vi "swerve math.vi"() -> ()   [LabVIEW 2020]
panel:
  out "Back Right":cluster{"X":dbl, "Y":dbl}[](graph)
  out "Back Left":cluster{"X":dbl, "Y":dbl}[](graph)
  out "Front Right":cluster{"X":dbl, "Y":dbl}[](graph)
  in  "RCW":dbl(slide) scale=-1.0..1.0
  in  "STR":dbl(slide) scale=-1.0..1.0
  in  "FWD":dbl(slide) scale=-1.0..1.0
  out "Front Left":cluster{"X":dbl, "Y":dbl}[](graph)
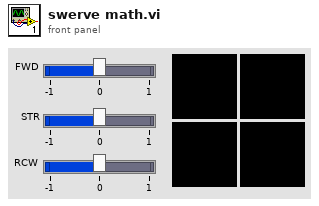
[diagram p1: front panel]
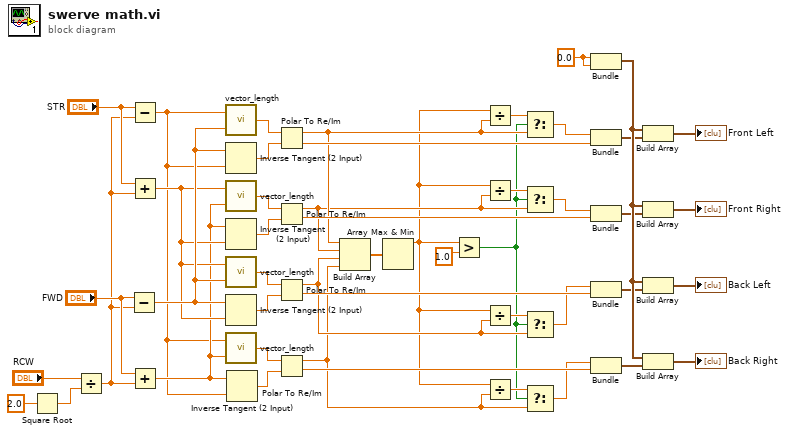
[diagram p0: block diagram]
diagram:
  w26 = 0.0 ("x")
  n1 = Square Root(x=2.0) -> (sqrt(x)=w48:dbl)
  n2 = Divide(x="RCW", y=w48) -> (x/y=w43:dbl)
  n3 = Subtract(x="FWD", y=w43) -> (x-y=w42:dbl)
  n4 = Subtract(x="STR", y=w43) -> (x-y=w39:dbl)
  n5 = Add(x="STR", y=w43) -> (x+y=w41:dbl)
  n6 = Add(x="FWD", y=w43) -> (x+y=w40:dbl)
  n7 = call "vector_length.vi"("v_y"=w42, "v_x"=w39) -> ("||v||"=w37:dbl)
  n8 = Inverse Tangent (2 Input)(1:w39, 2:w42) -> (0:w38:dbl)
  n9 = call "vector_length.vi"("v_y"=w40, "v_x"=w41) -> ("||v||"=w36:dbl)
  n10 = Inverse Tangent (2 Input)(1:w41, 2:w40) -> (0:w35:dbl)
  n11 = call "vector_length.vi"("v_y"=w42, "v_x"=w41) -> ("||v||"=w34:dbl)
  n12 = Inverse Tangent (2 Input)(1:w41, 2:w42) -> (0:w33:dbl)
  n13 = call "vector_length.vi"("v_y"=w40, "v_x"=w39) -> ("||v||"=w32:dbl)
  n14 = Inverse Tangent (2 Input)(1:w39, 2:w40) -> (0:w31:dbl)
  n15 = Polar To Re/Im(2:w38, 3:w37) -> (0:w30:dbl, 1:w17:dbl)
  n16 = Polar To Re/Im(2:w35, 3:w36) -> (0:w29:dbl, 1:w15:dbl)
  n17 = Polar To Re/Im(2:w33, 3:w34) -> (0:w28:dbl, 1:w13:dbl)
  n18 = Polar To Re/Im(2:w31, 3:w32) -> (0:w27:dbl, 1:w11:dbl)
  n19 = Build Array(w17, w15, w13, w11) -> (w20:dbl[])
  n20 = Array Max & Min(array=w20) -> (max value=w10:dbl)  [unwired: 3 out]
  n21 = Greater?(x=w10, y=1.0) -> (0:w5:bool)
  n22 = Divide(x=w10, y=w17) -> (x/y=w18:dbl)
  n23 = Divide(x=w10, y=w15) -> (x/y=w16:dbl)
  n24 = Divide(x=w10, y=w13) -> (x/y=w14:dbl)
  n25 = Divide(x=w10, y=w11) -> (x/y=w12:dbl)
  n26 = Select(t=w18, s=w5, f=w17) -> (s? t:f=w9:dbl)
  n27 = Select(t=w16, s=w5, f=w15) -> (s? t:f=w8:dbl)
  n28 = Select(t=w14, s=w5, f=w13) -> (s? t:f=w7:dbl)
  n29 = Select(t=w12, s=w5, f=w11) -> (s? t:f=w6:dbl)
  n30 = Bundle("x"=w26, "x"=w26) -> (w25:cluster{"x":dbl, "x":dbl})  [unwired: 1 in]
  n31 = Bundle(w9, w30) -> (w4:cluster{dbl, dbl})  [unwired: 1 in]
  n32 = Bundle(w8, w29) -> (w3:cluster{dbl, dbl})  [unwired: 1 in]
  n33 = Bundle(w7, w28) -> (w2:cluster{dbl, dbl})  [unwired: 1 in]
  n34 = Bundle(w6, w27) -> (w1:cluster{dbl, dbl})  [unwired: 1 in]
  n35 = Build Array(w25, w4) -> (→"Front Left":cluster{"x":dbl, "x":dbl}[])
  n36 = Build Array(w25, w3) -> (→"Front Right":cluster{"x":dbl, "x":dbl}[])
  n37 = Build Array(w25, w2) -> (→"Back Left":cluster{"x":dbl, "x":dbl}[])
  n38 = Build Array(w25, w1) -> (→"Back Right":cluster{"x":dbl, "x":dbl}[])
